vi "ReadU16Tiff_withtext.vi"(0 "file path":path, 1 "error in":errorcluster) -> (2 "I16 pixmap":u16[][](array[numeric]), 3 "string":string, 4 "error out":errorcluster)   [LabVIEW 2011]
uses:
  TiffModules/ReadTiffPage_U16_text_res.vi
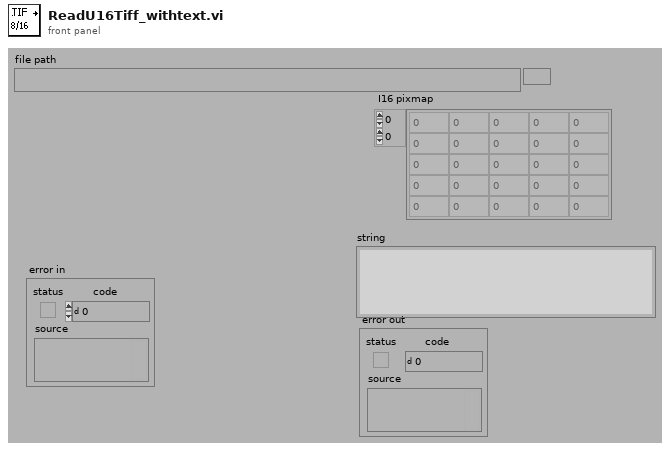
[diagram p1: front panel]
types:
  T1 = cluster{"Tiff refnum":refnum<file>, "BigTiff,Endian":u16}
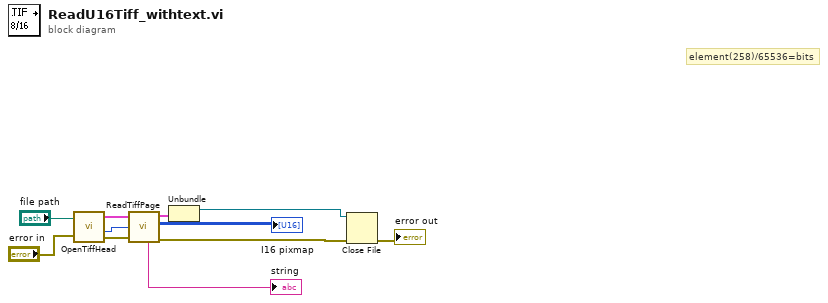
[diagram p0: block diagram]
diagram:
  # "element(258)/65536=bits"
  n1 = call "OpenTiffHead.vi"("file path"="file path", "error in"="error in") -> ("TIFF file"=w8:T1, "first Diroffset"=w6:u64, "error out"=w7:errorcluster)  [unwired: 1 out]
  n2 = call-poly "ReadTiffPage.vi"("TIFF file"=w8, "IFDoffset"=w6, "error in"=w7) -> ("TIFF file out"=w3:T1, "16-bit pixmap"=→"I16 pixmap":u16[][], "string"=→"string":string, "error out"=w2:errorcluster)  [unwired: 4 out]
  n3 = Unbundle(w3) -> ("Tiff refnum"=w1:refnum<file>)  [unwired: 1 out]
  n4 = Close File(refnum=w1, error in=w2) -> (error out=→"error out":errorcluster)  [unwired: 1 out]
